vi "openbci_parse_eeg_data.vi"(10 "Gain (24x)":T1=enum."24x", 11 "string_eeg_data":string) -> (3 "eeg_data":dbl[](array[numeric]))   [LabVIEW 2013]
doc: "For the EEG data values, data is transfered as a 24-bit integer (native format used by the ADS1299 EEG chip) that is at the core of the OpenBCI board."
uses:
  Comm Protocol/Control Def/gain_ADS1299.ctl
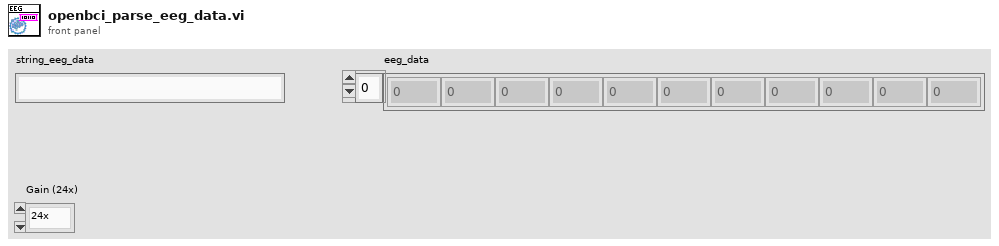
[diagram p1: front panel]
types:
  T1 = typedef "gain_ADS1299.ctl" = enum16{"1x", "2x", "4x", "8x", "16x", "24x"}
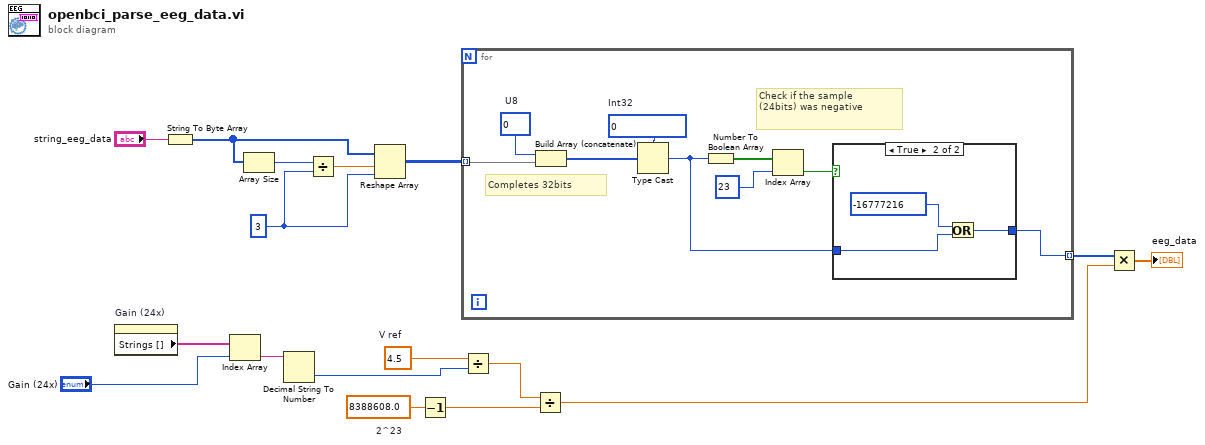
[diagram p0: block diagram]
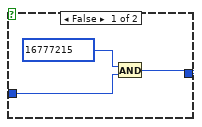
[diagram p2: hidden frame]
diagram:
  w9 = 8388608.0  # 2^23
  w10 = 4.5  # V ref
  w14 = 3 ("dimension size")
  n1 = property on="Gain (24x)" class="Enum (strict)"() -> ("Strings []"=w4:string[])  [unwired: 2 in, 2 out]
  n2 = String To Byte Array(string="string_eeg_data") -> (unsigned byte array=w16:u8[])
  n3 = Index Array(array=w4, index="Gain (24x)") -> (element=w2:string)
  n4 = Array Size(array=w16) -> (size(s)=w15:i32)
  n5 = Decimal String To Number(string=w2) -> (number=w1:i32)  [unwired: 2 in, 1 out]
  n6 = Divide(x=w15, y=w14) -> (x/y=w13:dbl)
  n7 = Reshape Array(w16, w13, w14) -> (w12:u8[][])
  n8 = Decrement(x=w9) -> (x-1=w7:dbl)
  n9 = for {
    tunnel: w12 -> [w25] mode=indexing
    tunnel: [w18] -> w11 mode=indexing
    w19 = 0  # Int32
    w26 = u8 0  # U8
    # "Check if the sample\n(24bits) was negative"
    # "Completes 32bits"
    n10 = Build Array (concatenate)(w26, w25) -> (w24:u8[])
    n11 = Type Cast(type=w19, x=w24) -> (*(type *) &x=w20:i32)
    n12 = Number To Boolean Array(number=w20) -> (Boolean array=w21:bool[])
    n13 = Index Array(array=w21, index=23) -> (element=w22:bool)
    n14 = case shown="True" w22 {
      tunnel: w20 -> [w28 w31]
      tunnel: [w27 w30] -> w18
      frame False {
        n15 = And(x=16777215 ("dimension size"), y=w28) -> (x .and. y?=w27:i32)
      }
      frame True {
        n16 = Or(x=-16777216 ("dimension size"), y=w31) -> (x .or. y?=w30:i32)
      }
    }
  }
  n17 = Divide(x=w10, y=w1) -> (x/y=w8:dbl)
  n18 = Divide(x=w8, y=w7) -> (x/y=w6:dbl)
  n19 = Multiply(x=w11, y=w6) -> (x*y=→"eeg_data":dbl[])
